vi "Live_Plotter_main.vi"() -> ()   [LabVIEW 2017]
uses:
  Controls/Plotter_Parameter_List_Record.ctl
  Classes/ADCP.lvclass
  Controls/Plotter_Globals.ctl
  Controls/Plotter_Queues.ctl
  Controls/Plotter_Queue_Command_and_Data.ctl
  Controls/Plotter_Commands.ctl
  Controls/Plotter_UI_Plot_Commands.ctl
panel:
  in  "ADCP.lvclass":refnum<class "ADCP.lvclass">
  in  "Exit Application":bool
  in  "Enable/Disable node connection":bool caption="Enable/Disable node"
  out "Receive Parameter List":T1[](array[typedef])
  out "Run Duration (ms)":u32
  in  "Transmit Parameter To Node":bool
  in  "Transmit Parameter Value":string
  in  "Transmit Parameter":string(combo)
  in  "Remove Parameter":bool caption="Remove"
  in  "Add Parameter":bool caption="Add"
  in  "Plot Parameter":string(combo)
  in  "Set Log File Name":bool
  in  "Session Name":string
  in  "Load Symbol File":bool
  in  "Symbol File Path":path=path "F:/Projects/ADCP/LabVIEW/Symbol Files/default.csv"
  in  "Connect/Disconnect Serial Port":bool
  in  "Baud Rate":u32
  in  "COM Port":refnum<visa-resource-name>="COM12"
  out "Plot":cluster{"Time (ms)":dbl[], "Values":dbl[]}[](graph)
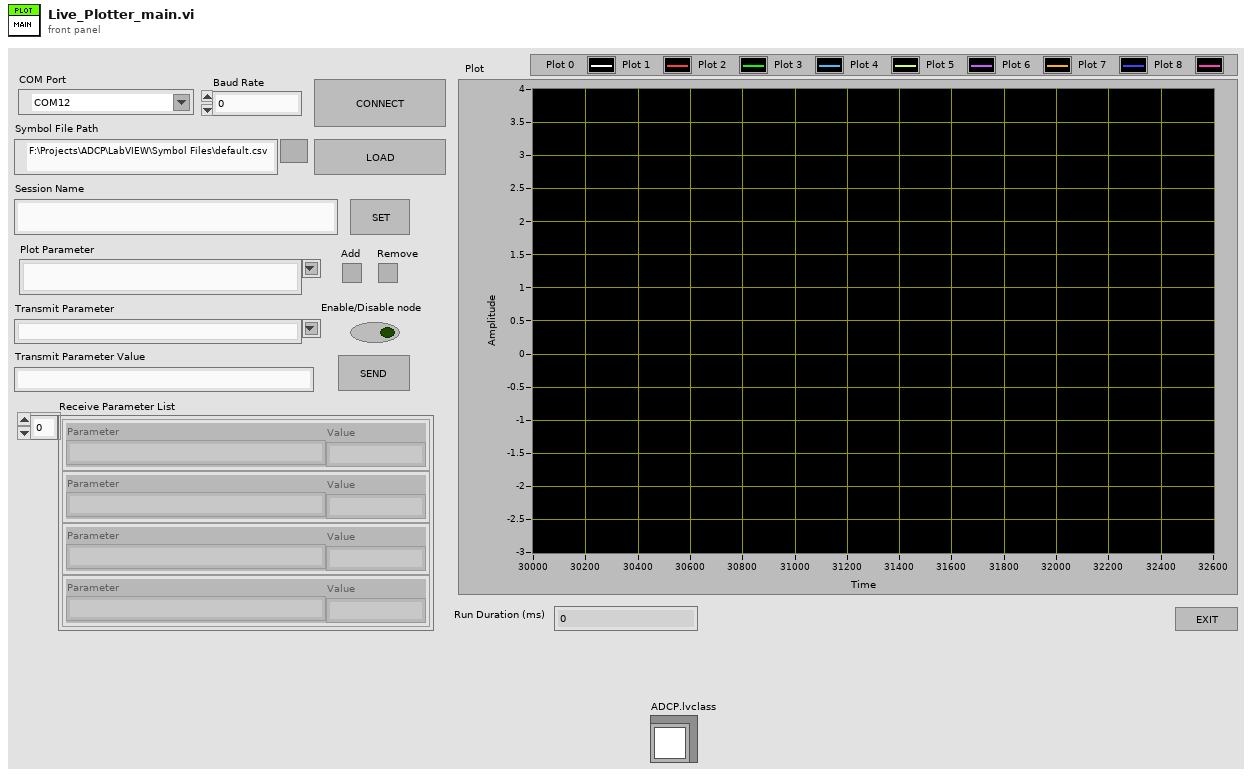
[diagram p1: front panel]
types:
  T1 = typedef "Plotter_Parameter_List_Record.ctl" = cluster{"Parameter":string, "Value":string}
  T2 = typedef "Plotter_UI_Plot_Commands.ctl" = enum16{"Initialize", "Update", "Clear"}
  T3 = typedef "Plotter_Globals.ctl" = cluster{"Enable/Disable node connection":refnum<vi>, "Receive Parameter List":refnum<vi>, "Run Duration (ms)":refnum<vi>, "Transmit Parameter Value":refnum<vi>, "Transmit Parameter":refnum<vi>, "Remove Parameter":refnum<vi>, "Add Parameter":refnum<vi>, "Plot Parameter":refnum<vi>, "Session Name":refnum<vi>, "Symbol File Path":refnum<vi>, "Connect/Disconnect Serial Port":refnum<vi>, "Baud Rate":refnum<vi>, "COM Port":refnum<vi>, "Plot":refnum<vi>, "Transmit Parameter To Node":refnum<vi>, "Set Log File Name":refnum<vi>, "Load Symbol File":refnum<vi>, "Exit Application":refnum<vi>, "ADCP":refnum<vi>, "Transmit Log File Path":refnum<vi>, "Receive Log File Path":refnum<vi>, "Queues":T4}
  T4 = typedef "Plotter_Queues.ctl" = cluster{"Continuous Receiver":refnum<queue>, "Receiver - Log File":refnum<queue>, "Receiver - Plotter Parameter List":refnum<queue>, "Write Parameter":refnum<queue>}
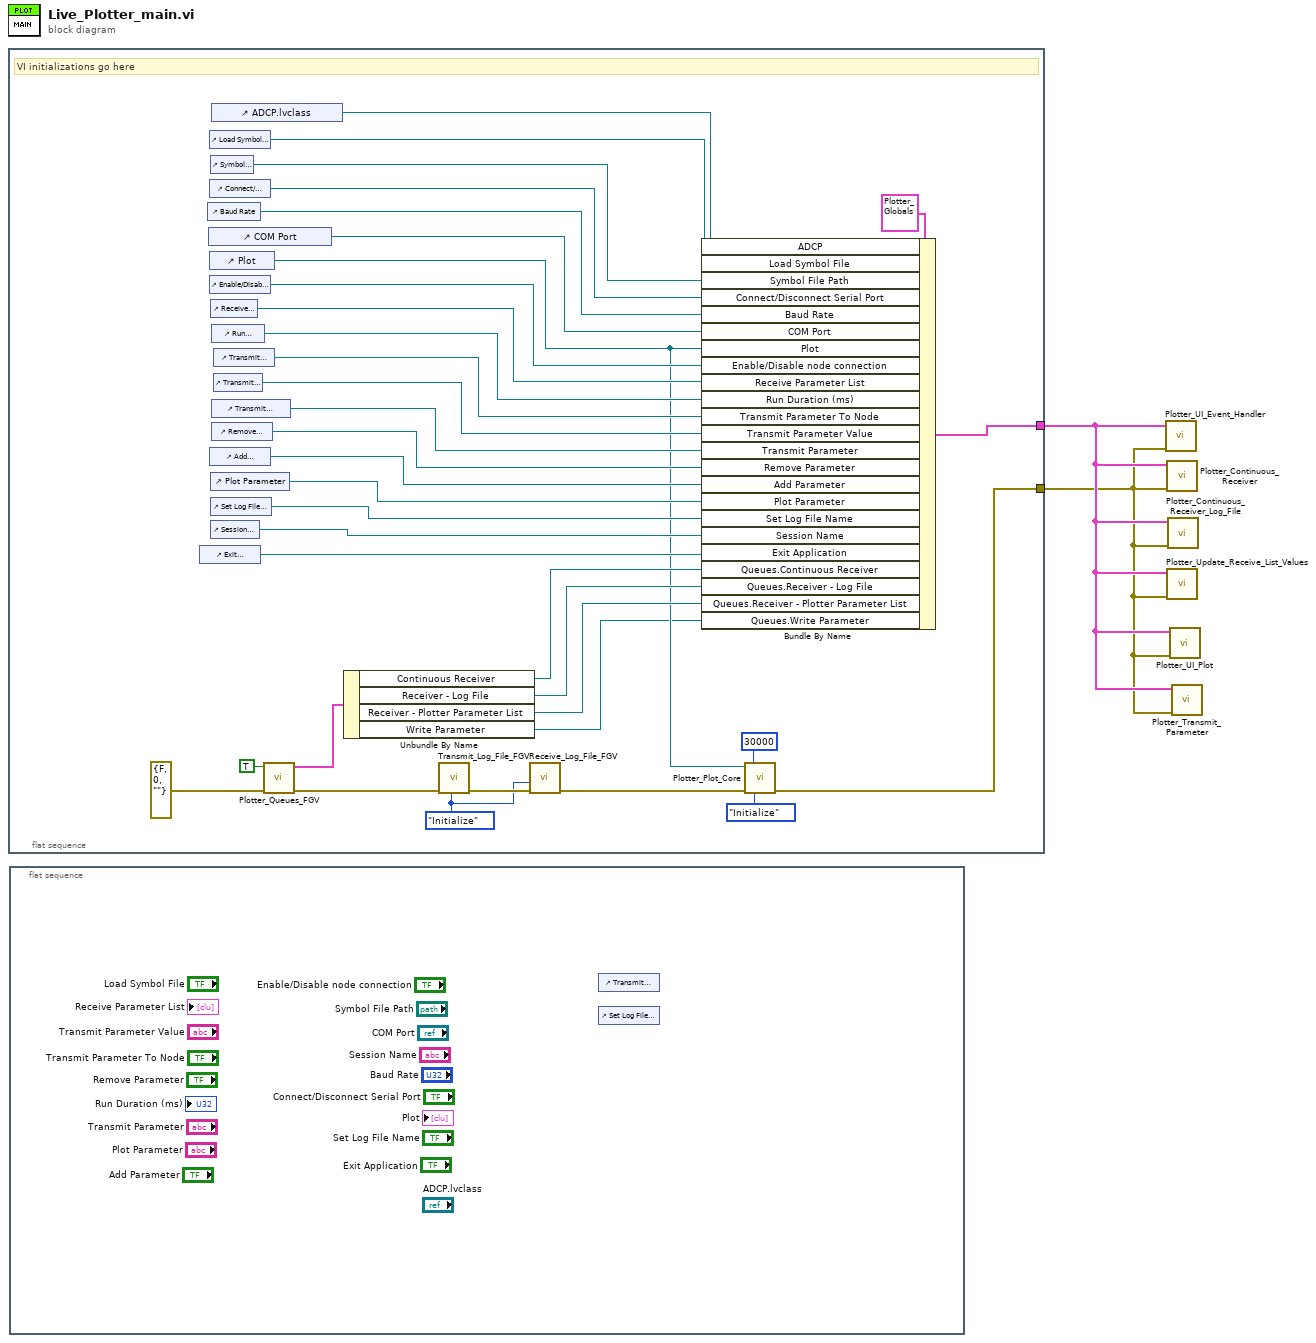
[diagram p0: block diagram]
diagram:
  n1 = flat-sequence {
    tunnel: [w20] -> w2
    tunnel: [w7] -> w1
    frame #0 {
      w10 = enum16{"Initialize", "Update", "Stop"}."Initialize" ("Command")
      # "VI initializations go here"
      n2 = control-ref of="Exit Application"() -> (w19:refnum<vi>)
      n3 = control-ref of="Baud Rate"() -> (w33:refnum<vi>)
      n4 = control-ref of="COM Port"() -> (w32:refnum<vi>)
      n5 = control-ref of="Load Symbol File"() -> (w37:refnum<vi>)
      n6 = control-ref of="Connect/Disconnect Serial Port"() -> (w34:refnum<vi>)
      n7 = control-ref of="Plot"() -> (w5:refnum<vi>)
      n8 = control-ref of="Enable/Disable node connection"() -> (w31:refnum<vi>)
      n9 = control-ref of="Add Parameter"() -> (w24:refnum<vi>)
      n10 = control-ref of="Symbol File Path"() -> (w36:refnum<vi>)
      n11 = control-ref of="Receive Parameter List"() -> (w30:refnum<vi>)
      n12 = control-ref of="Plot Parameter"() -> (w23:refnum<vi>)
      n13 = control-ref of="Set Log File Name"() -> (w22:refnum<vi>)
      n14 = control-ref of="Session Name"() -> (w21:refnum<vi>)
      n15 = control-ref of="ADCP.lvclass"() -> (w18:refnum<vi>)
      n16 = control-ref of="Run Duration (ms)"() -> (w29:refnum<vi>)
      n17 = control-ref of="Transmit Parameter"() -> (w26:refnum<vi>)
      n18 = control-ref of="Remove Parameter"() -> (w25:refnum<vi>)
      n19 = control-ref of="Transmit Parameter To Node"() -> (w28:refnum<vi>)
      n20 = control-ref of="Transmit Parameter Value"() -> (w27:refnum<vi>)
      n21 = call "Plotter_Queues_FGV.vi"("error in (no error)"=errorcluster {"status"=FALSE, "code"=0, "source"=""} ("error constant"), "Initialize ?"=TRUE) -> ("error out"=w12:errorcluster, "Queues"=w15:T4)  [unwired: 8 in]
      n22 = Unbundle By Name(w15) -> ("Continuous Receiver"=w14:refnum<queue>, "Receiver - Log File"=w13:refnum<queue>, "Receiver - Plotter Parameter List"=w9:refnum<queue>, "Write Parameter"=w3:refnum<queue>)
      n23 = call "Transmit_Log_File_FGV.vi"("error in (no error)"=w12, "Command"=w10) -> ("error out"=w11:errorcluster)  [unwired: 8 in, 1 out]
      n24 = call "Receive_Log_File_FGV.vi"("error in (no error)"=w11, "Command"=w10) -> ("error out"=w8:errorcluster)  [unwired: 8 in, 1 out]
      n25 = Bundle By Name(cluster=T3 {"Enable/Disable node connection"=refnum, "Receive Parameter List"=refnum, "Run Duration (ms)"=refnum, "Transmit Parameter Value"=refnum, "Transmit Parameter"=refnum, "Remove Parameter"=refnum, "Add Parameter"=refnum, "Plot Parameter"=refnum, "Session Name"=refnum, "Symbol File Path"=refnum, "Connect/Disconnect Serial Port"=refnum, "Baud Rate"=refnum, "COM Port"=refnum, "Plot"=refnum, "Transmit Parameter To Node"=refnum, "Set Log File Name"=refnum, "Load Symbol File"=refnum, "Exit Application"=refnum, "ADCP"=refnum, "Transmit Log File Path"=refnum, "Receive Log File Path"=refnum, "Queues"={"Continuous Receiver"=refnum, "Receiver - Log File"=refnum, "Receiver - Plotter Parameter List"=refnum, "Write Parameter"=refnum}}, "ADCP"=w18, "Load Symbol File"=w37, "Symbol File Path"=w36, "Connect/Disconnect Serial Port"=w34, "Baud Rate"=w33, "COM Port"=w32, "Plot"=w5, "Enable/Disable node connection"=w31, "Receive Parameter List"=w30, "Run Duration (ms)"=w29, "Transmit Parameter To Node"=w28, "Transmit Parameter Value"=w27, "Transmit Parameter"=w26, "Remove Parameter"=w25, "Add Parameter"=w24, "Plot Parameter"=w23, "Set Log File Name"=w22, "Session Name"=w21, "Exit Application"=w19, "Queues.Continuous Receiver"=w14, "Queues.Receiver - Log File"=w13, "Queues.Receiver - Plotter Parameter List"=w9, "Queues.Write Parameter"=w3) -> (w20:T3)
      n26 = call "Plotter_Plot_Core.vi"("error in (no error)"=w8, "Refresh interval (ms)"=u32 30000, "Commands"=Plotter_UI_Plot_Commands."Initialize", "XY Graph"=w5) -> ("error out"=w7:errorcluster)  [unwired: 7 in]
    }
  }
  n27 = flat-sequence {
    frame #0 {
      n28 = control-ref of="Transmit Parameter To Node"() -> ()  [unwired: 1 out]
      n29 = control-ref of="Set Log File Name"() -> ()  [unwired: 1 out]
    }
  }
  n30 = call "Plotter_UI_Event_Handler.vi"("error in (no error)"=w1, "Globals"=w2) -> ()  [unwired: 9 in, 1 out]
  n31 = call "Plotter_Continuous_Receiver.vi"("error in (no error)"=w1, "Global Variables"=w2) -> ()  [unwired: 10 in]
  n32 = call "Plotter_Update_Receive_List_Values.vi"("error in (no error)"=w1, "Globals"=w2) -> ()  [unwired: 10 in]
  n33 = call "Plotter_Continuous_Receiver_Log_File.vi"("error in (no error)"=w1, "Globals"=w2) -> ()  [unwired: 10 in]
  n34 = call "Plotter_UI_Plot.vi"("error in (no error)"=w1, "Globals"=w2) -> ()  [unwired: 10 in]
  n35 = call "Plotter_Transmit_Parameter.vi"("error in (no error)"=w1, "Globals"=w2) -> ()  [unwired: 10 in]
